vi "DAQNavi Read (Counter 2D Count Value NChan NSamp).vi"(8 "error in (no error)":errorcluster, 9 "number of samples per channel to read":u32=10, 10 "timeout":dbl=10.0, 11 "task in":i32) -> (0 "error out":errorcluster, 2 "data":i32[][](array[numeric]), 3 "task out":i32)   [LabVIEW 2020]
uses:
  DAQNavi_LV.dll
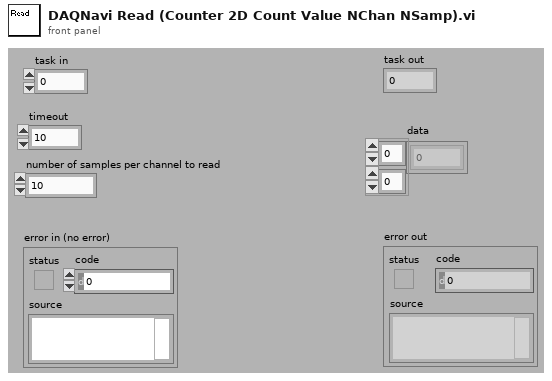
[diagram p1: front panel]
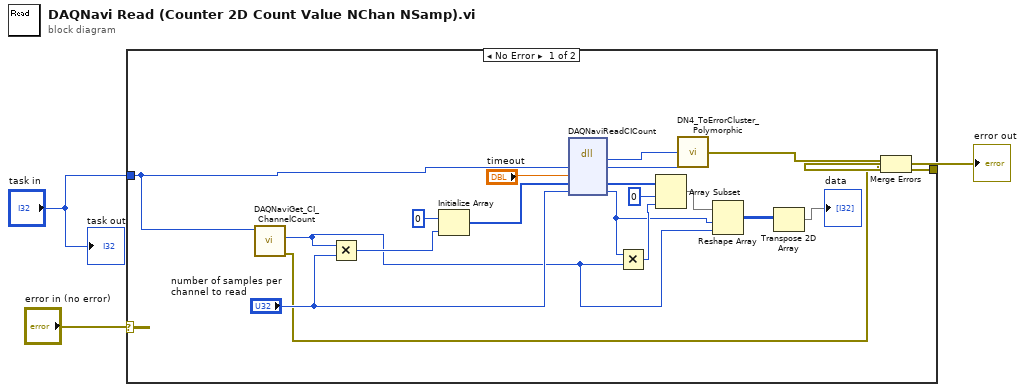
[diagram p0: block diagram]
diagram:
  n1 = case shown="No Error" "error in (no error)" {
    selector: "error in (no error)" -> [_ w23]
    tunnel: "task in" -> [w15 _]
    tunnel: [w12 w23] -> w1
    frame No Error {
      n2 = call "DAQNaviGet_CI_ChannelCount.vi"("task in"=w15) -> ("error out"=w10:errorcluster, "channel count"=w6:i32)  [unwired: 1 in, 8 out]
      n3 = Multiply(x=w6, y="number of samples per channel to read") -> (x*y=w13:u32)
      n4 = Initialize Array(0 ("element"), w13) -> (w17:i32[])
      n5 = dll-call lib="DAQNavi_LV.dll" fn="DAQNaviReadCICount"("taskID"=w15, "timeout"="timeout", "count"=w17, "samples"="number of samples per channel to read") -> ("return type"=w22:i32, "taskID"=w16:i32, "count"=w20:i32[], "samples"=w7:u32)  [unwired: 4 in, 2 out]
      n6 = Multiply(x=w7, y=w6) -> (x*y=w9:u32)
      n7 = Array Subset(array=w20, index=0, length=w9) -> (w8:i32[])
      n8 = call "DN4_ToErrorCluster_Polymorphic.vi"("task id"=w16, "error code"=w22) -> ("error out"=w11:errorcluster)  [unwired: 3 out]
      n9 = Reshape Array(w8, w7, w6) -> (w5:i32[][])
      n10 = Transpose 2D Array(2D array=w5) -> (transposed array=→"data":i32[][])
      n11 = Merge Errors(w11, w10) -> (w12:errorcluster)
    }
    frame Error {
    }
  }
  "error out" <- w1
  "task out" <- "task in"
